vi "CheckForEmpty.vi"(11 "Strings [] in":string[](array[string])) -> (3 "Strings [] out":string[](array[string]))   [LabVIEW 2022 SP3]
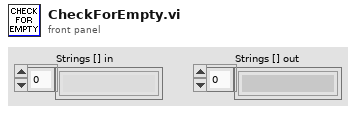
[diagram p1: front panel]
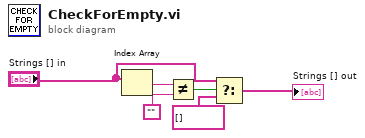
[diagram p0: block diagram]
diagram:
  n1 = Index Array(array="Strings [] in") -> (element=w1:string)  [unwired: 1 in]
  n2 = Not Equal?(x=w1, y="") -> (x != y?=w3:bool)
  n3 = Select(t="Strings [] in", s=w3, f=string[] []) -> (s? t:f=→"Strings [] out":string[])
